vi "GetParameterValue(I16).vi"(8 "error in (no error)":errorcluster, 10 "hcam in":i16, 11 "Param ID (Ring)":T1) -> (0 "error out":errorcluster, 2 "ParameterValue":i16, 3 "hcam out":i16)   [LabVIEW 2013]
uses:
  PARAM_ID_TypDef.ctl
  getParameterValue.vi
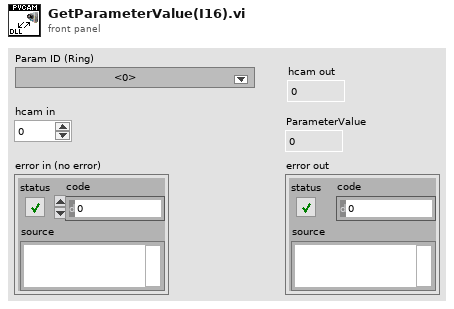
[diagram p1: front panel]
types:
  T1 = typedef "PARAM_ID_TypDef.ctl" = u32
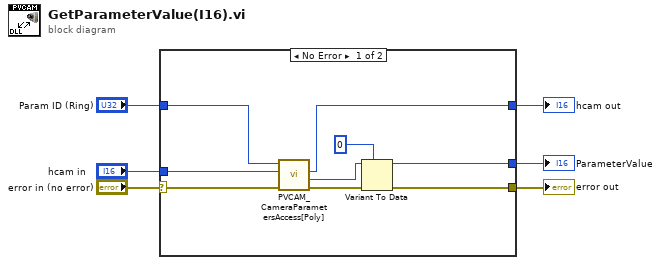
[diagram p0: block diagram]
diagram:
  n1 = case shown="No Error" "error in (no error)" {
    selector: "error in (no error)" -> [w7 w17]
    tunnel: [w15 w17] -> w6
    tunnel: [w14 _] -> w5
    tunnel: "hcam in" -> [w10 w16]
    tunnel: "Param ID (Ring)" -> [w9 _]
    tunnel: [w8 w16] -> w2
    frame No Error {
      n2 = call-poly "PVCAM_CameraParametersAccess[Poly].vi"("error in (no error)"=w7, "hcam"=w10, "Param ID (Ring)"=w9) -> ("error out"=w11:errorcluster, "param_value"=w12:variant, "hcam out"=w8:i16)  [unwired: 4 in, 2 out]
      n3 = Variant To Data(error in=w11, type=i16 0, Variant=w12) -> (data=w14:i16, error out=w15:errorcluster)
    }
    frame Error {
    }
  }
  "error out" <- w6
  "ParameterValue" <- w5
  "hcam out" <- w2
